vi "Destroy.vi"(8 "Error In":errorcluster, 11 "LabSSH2":refnum<class "Context.lvclass">) -> (0 "Error Out":errorcluster)   [LabVIEW 2017, in "LabSSH2.lvlib" / "Context.lvclass"]
uses:
  Context.lvclass
  Context.lvclass/Context.ctl
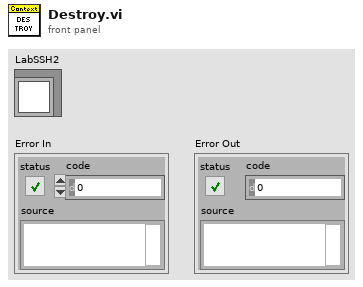
[diagram p1: front panel]
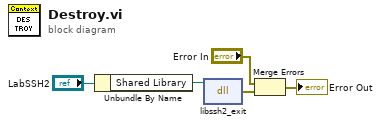
[diagram p0: block diagram]
diagram:
  n1 = Unbundle By Name("LabSSH2") -> ("Shared Library"=w3:path)
  n2 = dll-call lib="C:/Program Files/libssh2/bin/libssh2.dll" fn="libssh2_exit"(path in=w3) -> (error out=w5:errorcluster)  [unwired: 3 in, 1 out]
  n3 = Merge Errors("Error In", w5) -> (→"Error Out":errorcluster)
